vi "Short Relative - Copy.vi"(0 "Wanted Angle":dbl, 1 "Current Angle":dbl) -> (7 "Change in angle":dbl, 8 "Cluster":T1)   [LabVIEW 2020]
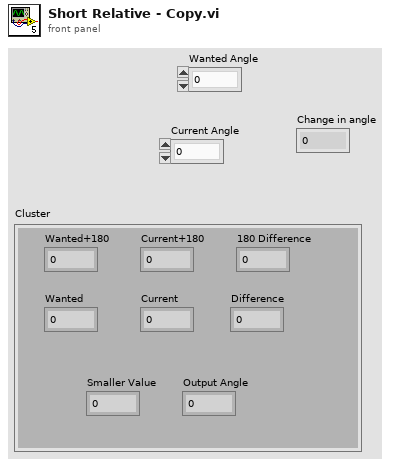
[diagram p1: front panel]
types:
  T1 = cluster{"Wanted+180":dbl, "Current+180":dbl, "180 Difference":dbl, "Wanted":dbl, "Current":dbl, "Difference":dbl, "Smaller Value":dbl, "Output Angle":dbl}
  T2 = cluster{dbl, dbl, dbl, "Wanted Angle":dbl, "Current Angle":dbl, dbl, dbl, dbl}
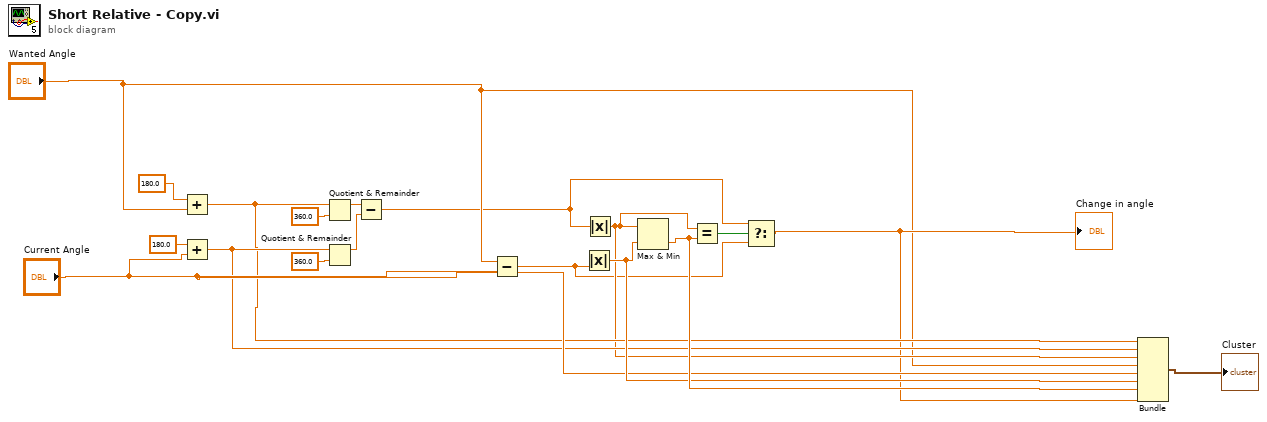
[diagram p0: block diagram]
diagram:
  n1 = Add(x=180.0, y="Wanted Angle") -> (x+y=w13:dbl)
  n2 = Add(x=180.0, y="Current Angle") -> (x+y=w14:dbl)
  n3 = Quotient & Remainder(x=w13, y=360.0) -> (x-y*floor(x/y)=w5:dbl)  [unwired: 1 out]
  n4 = Quotient & Remainder(x=w14, y=360.0) -> (x-y*floor(x/y)=w4:dbl)  [unwired: 1 out]
  n5 = Subtract(x=w5, y=w4) -> (x-y=w2:dbl)
  n6 = Subtract(x="Wanted Angle", y="Current Angle") -> (x-y=w1:dbl)
  n7 = Absolute Value(x=w1) -> (abs(x)=w16:dbl)
  n8 = Absolute Value(x=w2) -> (abs(x)=w12:dbl)
  n9 = Max & Min(x=w12, y=w16) -> (min(x,y)=w17:dbl)  [unwired: 1 out]
  n10 = Equal?(x=w12, y=w17) -> (x = y?=w3:bool)
  n11 = Select(t=w2, s=w3, f=w1) -> (s? t:f=w11:dbl)
  "Change in angle" <- w11
  n12 = Bundle(w13, w14, w12, "Wanted Angle"="Wanted Angle", "Current Angle"="Current Angle", w16, w17, w11) -> (→"Cluster":T2)  [unwired: 1 in]
